vi "fgv_udp_remote1.vi"(7 "cmd":T2, 8 "error in":errorcluster) -> (0 "error out":errorcluster, 3 "queue out":refnum<queue>)   [LabVIEW 2019]
uses:
  Ctrl/fgv_q.ctl
  Ctrl/q_data-type.ctl
panel:
  in  "data":T1
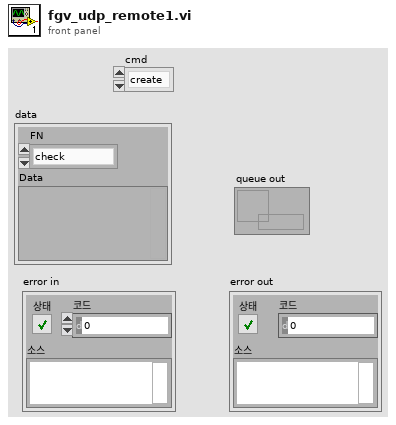
[diagram p1: front panel]
types:
  T1 = typedef "q_data-type.ctl" = cluster{"FN":enum16{"check", "run"}, "Data":variant}
  T2 = typedef "fgv_q.ctl" = enum16{"create", "read", "write", "close"}
  T3 = cluster{"FN":enum16{"check", "run"}, "Data":variant}
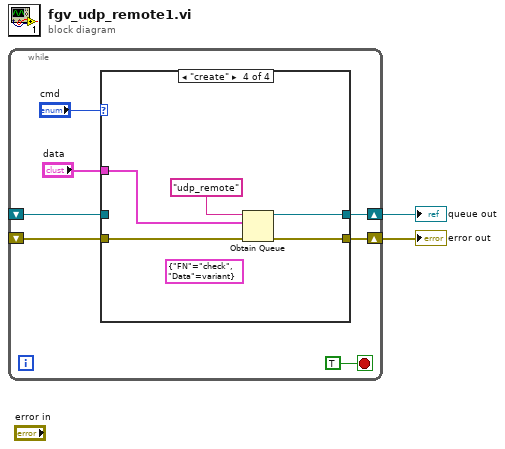
[diagram p0: block diagram]
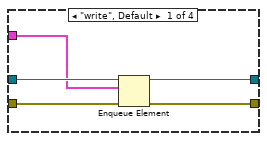
[diagram p2: hidden frame]
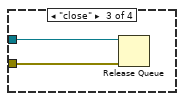
[diagram p4: hidden frame]
diagram:
  n1 = while {
    shift-right: [w5] -> w2
    shift-left: _ -> [w4]
    shift-right: [w6] -> w1
    shift-left: _ -> [w7]
    stop <- TRUE stop-if-true
    n2 = case shown="\"create\"" "cmd" {
      tunnel: w7 -> [w13 w16 w18 w23]
      tunnel: [w14 w16 _ w22] -> w6
      tunnel: [w12 w15 _ w21] -> w5
      tunnel: w4 -> [w11 w15 w17 _]
      tunnel: "data" -> [w10 _ _ w19]
      frame "write", Default {
        n3 = Enqueue Element(queue=w11, element=w10, error in (no error)=w13) -> (queue out=w12:refnum<queue>, error out=w14:errorcluster)  [unwired: 1 in, 1 out]
      }
      frame "read" {
      }
      frame "close" {
        n4 = Release Queue(queue=w17, error in (no error)=w18) -> ()  [unwired: 1 in, 3 out]
      }
      frame "create" {
        (unwired) T3 {"FN"=enum."check", "Data"=variant} ("element")
        n5 = Obtain Queue(name (unnamed)="udp_remote" ("이름(이름없음)"), element data type=w19, error in (no error)=w23) -> (queue out=w21:refnum<queue>, error out=w22:errorcluster)  [unwired: 2 in, 1 out]
      }
    }
  }
  "queue out" <- w2
  "error out" <- w1
